vi "Comm Fail.vi"(6 "CRC Match":bool, 8 "error in (no error)":errorcluster) -> (0 "error out":errorcluster)   [LabVIEW 2014, in "ALPHA5 RS485.lvlib"]
uses:
  ALPHA5 RS485.lvlib
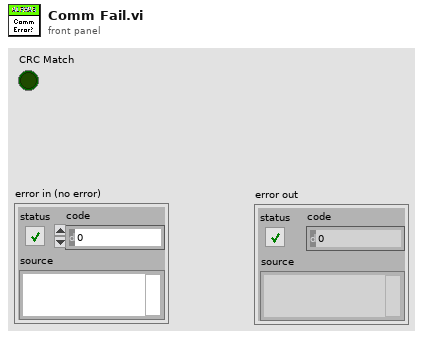
[diagram p1: front panel]
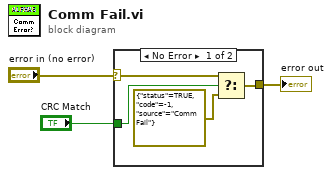
[diagram p0: block diagram]
diagram:
  n1 = case shown="No Error" "error in (no error)" {
    selector: "error in (no error)" -> [w6 w8]
    tunnel: "CRC Match" -> [w7 _]
    tunnel: [w4 w8] -> w1
    frame No Error {
      n2 = Select(t=w6, s=w7, f=errorcluster {"status"=TRUE, "code"=-1, "source"="Comm Fail"}) -> (s? t:f=w4:errorcluster)
    }
    frame Error {
    }
  }
  "error out" <- w1
